vi "Constructor.vi"(8 "error in (no error)":errorcluster, 11 "Mozzarella in":refnum<class "Mozzarella.lvclass">) -> (0 "error out":errorcluster, 2 "Ingredients":string, 3 "Mozzarella out":refnum<class "Mozzarella.lvclass">)   [LabVIEW 2013, in "Mozzarella.lvclass"]
uses:
  Mozzarella.lvclass
panel:
  # "我是意大利乾酪"
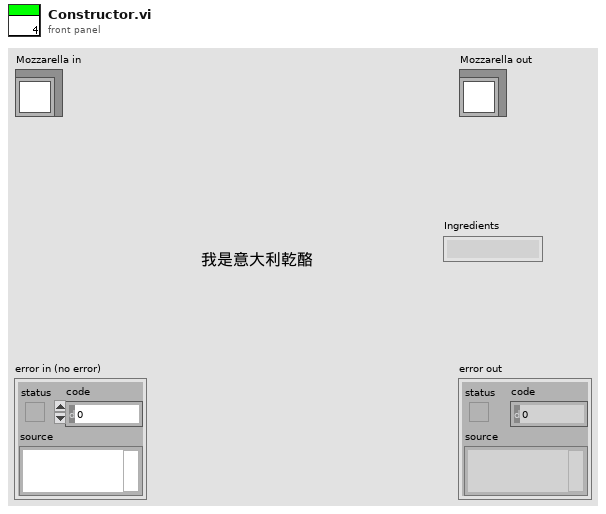
[diagram p1: front panel]
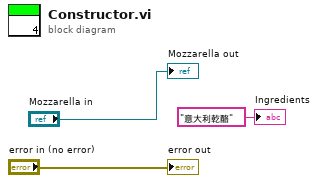
[diagram p0: block diagram]
diagram:
  "error out" <- "error in (no error)"
  "Mozzarella out" <- "Mozzarella in"
  "Ingredients" <- "意大利乾酪" ("Ingredients")
